vi "Flatten Value.vi"(8 "error in (no error)":errorcluster, 11 "Boolean in":refnum<class "Boolean.lvclass">) -> (0 "error out":errorcluster, 2 "Value":string, 3 "Boolean out":refnum<class "Boolean.lvclass">)   [LabVIEW 2019, in "Boolean.lvclass"]
uses:
  <vilib>/gpm_packages/@cs/data-type-serializer/source/Boolean/Boolean.lvclass
  <vilib>/gpm_packages/@cs/data-type-serializer/source/Boolean/Boolean.lvclass/Boolean.ctl
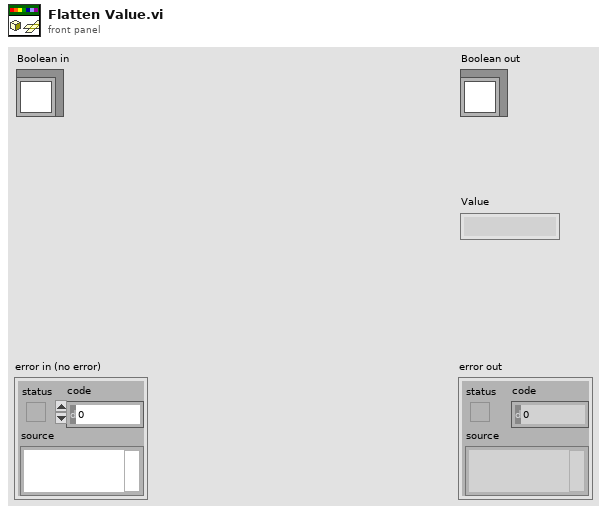
[diagram p1: front panel]
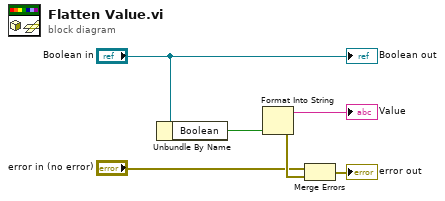
[diagram p0: block diagram]
diagram:
  n1 = Unbundle By Name("Boolean in") -> ("Boolean"=w5:bool)
  n2 = Format Into String(w5) -> (resulting string=→"Value":string, error out=w3:errorcluster)  [unwired: 3 in]
  n3 = Merge Errors("error in (no error)", w3) -> (→"error out":errorcluster)
  "Boolean out" <- "Boolean in"
